vi "_getWaveformContext - Copy.vi"(8 "error in":errorcluster, 11 "Context":string[](array[string])) -> (0 "error out":errorcluster, 2 "Values":variant[][](array[variant]), 3 "Names":string[][](array[string]))   [LabVIEW 2019]
uses:
  <vilib>/JDP Science/JSONtext/JSONtext.lvlib
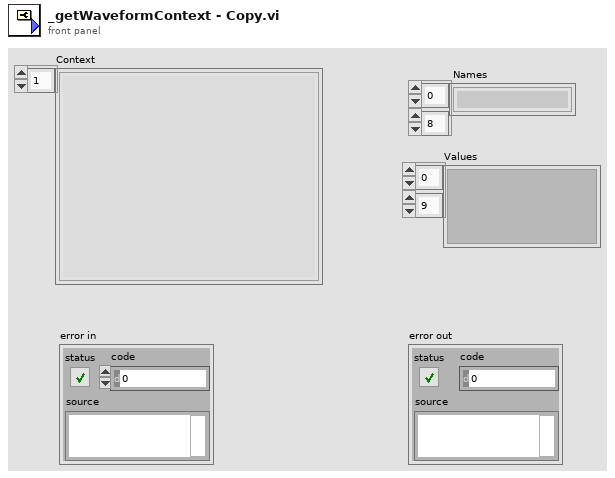
[diagram p1: front panel]
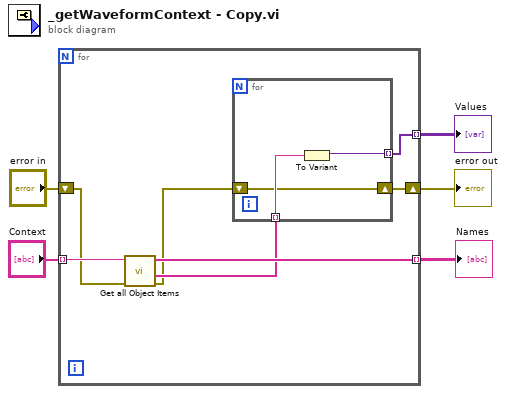
[diagram p0: block diagram]
diagram:
  n1 = for {
    tunnel: "Context" -> [w12] mode=indexing
    tunnel: [w10] -> w4 mode=indexing
    shift-right: [w11] -> w2
    shift-left: "error in" -> [w8]
    tunnel: [w6] -> w1 mode=indexing
    n2 = call <vilib>:"Get all Object Items.vi"("error in (no error)"=w8, "JSON"=w12) -> ("error out"=w7:errorcluster, "<JSON>"=w9:string[], "Item Names"=w10:string[])  [unwired: 6 in, 1 out]
    n3 = for {
      shift-right: [w13] -> w11
      shift-left: w7 -> [w13]
      tunnel: w9 -> [w15] mode=indexing
      tunnel: [w14] -> w6 mode=indexing
      n4 = To Variant(anything=w15) -> (Variant=w14:variant)
    }
  }
  "Names" <- w4
  "error out" <- w2
  "Values" <- w1
